vi "Update Config.vi"(8 "error in (no error)":errorcluster, 10 "Config":T1, 11 "HistorianCharting in":refnum<class "HistorianCharting.lvclass">) -> (0 "error out":errorcluster, 3 "HistorianCharting out":refnum<class "HistorianCharting.lvclass">)   [LabVIEW 2020, in "VolatusGUIElements.lvlib" / "HistorianCharting.lvclass"]
uses:
  HistorianCharting.lvclass
  HistorianCharting.lvclass/HistorianCharting.ctl
  Volatus/MessageQ/MessageQ.lvclass
  VolatusGUI/Historian Charting Manager/X-Axis Type.ctl
  VolatusGUI/Historian Charting Manager/Historian Charting Manager.lvclass
  VolatusGUI/Historian Charting Manager/Scale.ctl
  VolatusGUI/Historian Charting Manager/Plot Config.ctl
  VolatusGUI/Historian Charting Manager/Plot Group Config.ctl
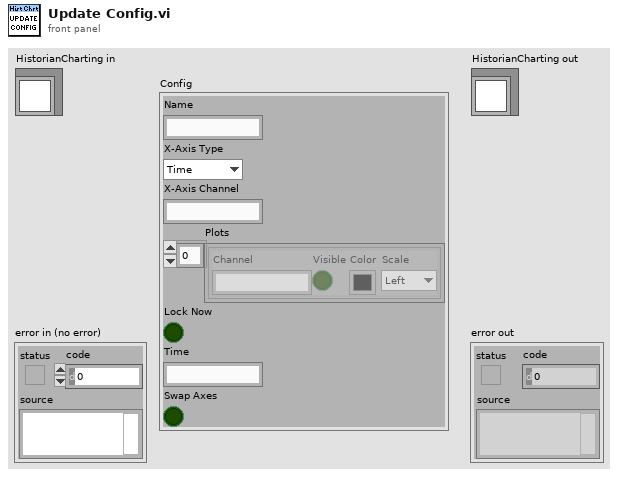
[diagram p1: front panel]
types:
  T1 = typedef "VolatusGUI.lvlib/Historian Charting Manager.lvclass/Plot Group Config.ctl" = cluster{"Name":string, "X-Axis Type":T2, "X-Axis Channel":string, "Plots":T3[], "Lock Now":bool, "Time":string, "Swap Axes":bool}
  T2 = typedef "VolatusGUI.lvlib/Historian Charting Manager.lvclass/X-Axis Type.ctl" = enum16{"Time", "Channel"}
  T3 = typedef "VolatusGUI.lvlib/Historian Charting Manager.lvclass/Plot Config.ctl" = cluster{"Channel":string, "Visible":bool, "Color":u32, "Scale":T4}
  T4 = typedef "VolatusGUI.lvlib/Historian Charting Manager.lvclass/Scale.ctl" = enum16{"Left", "Right"}
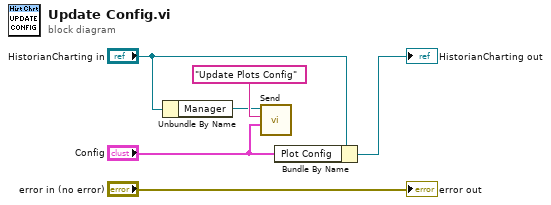
[diagram p0: block diagram]
diagram:
  n1 = Unbundle By Name("HistorianCharting in") -> ("Manager"=w3:refnum<class "MessageQ.lvclass">)
  n2 = call "Send.vi"("Data"="Config", "ID"="Update Plots Config", "MessageQ in"=w3) -> ()  [unwired: 7 in, 2 out]
  n3 = Bundle By Name(cluster="HistorianCharting in", "Plot Config"="Config") -> (→"HistorianCharting out":refnum<class "HistorianCharting.lvclass">)
  "error out" <- "error in (no error)"
